vi "PH_StatusHandler.set GUI Refs.vi"(0 "i ref in":refnum<vi>, 1 "Class":string, 2 "GUI Ref":refnum<vi>, 3 "Blinking (false)":bool, 4 "Tip Strip":string="N/A", 5 "error in (no error)":errorcluster) -> (14 "i ref out":refnum<vi>, 19 "error out":errorcluster)   [LabVIEW 2014, in "PH_StatusHandler.lvlib"]
doc: "By this VI the GUI refs are stored to own attributes."
uses:
  PH_StatusHandler.lvlib
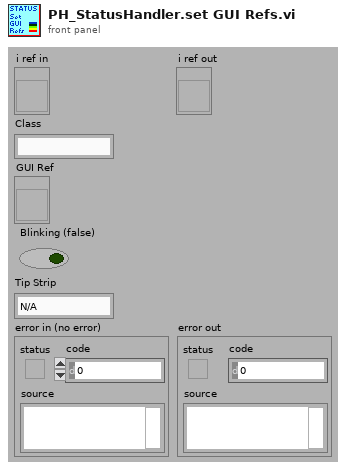
[diagram p1: front panel]
types:
  T1 = typedef "PH_StatusHandler.lvlib/PH_StatusHandler.i attribute.ctl" = cluster{"GUI Ref":refnum<vi>, "Value":T2, "Service ID":i32}
  T2 = typedef "PH_StatusHandler.lvlib/PH_StatusHandler.Status.ctl" = i16
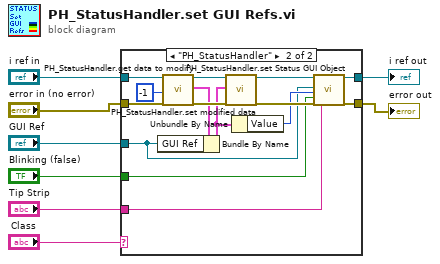
[diagram p0: block diagram]
diagram:
  n1 = case shown="\"PH_StatusHandler\"" "Class" {
    tunnel: "i ref in" -> [w10 w24]
    tunnel: "error in (no error)" -> [w9 w23]
    tunnel: "GUI Ref" -> [_ w13]
    tunnel: [w10 w18] -> w5
    tunnel: [w9 w16] -> w4
    tunnel: "Blinking (false)" -> [_ w12]
    tunnel: "Tip Strip" -> [_ w11]
    frame Default {
    }
    frame "PH_StatusHandler" {
      n2 = call "PH_StatusHandler.get data to modify.vi"("i ref in"=w24, "ms timeout (10000)"=-1, "error in (no error)"=w23) -> ("i ref out"=w20:refnum<vi>, "i attribute"=w21:T1, "error out"=w22:errorcluster)  [unwired: 13 in, 1 out]
      n3 = Bundle By Name(cluster=w21, "GUI Ref"=w13) -> (w15:T1)
      n4 = call "PH_StatusHandler.set modified data.vi"("i ref in"=w20, "i attribute"=w15, "error in (no error)"=w22) -> ("i ref out"=w18:refnum<vi>, "error out"=w17:errorcluster)  [unwired: 15 in]
      n5 = Unbundle By Name(w15) -> ("Value"=w14:T2)
      n6 = call "PH_StatusHandler.set Status GUI Object.vi"("PH Status Ref"=w13, "Value"=w14, "Blinking (false)"=w12, "error in (no error)"=w17, "Tip Strip"=w11) -> ("error out"=w16:errorcluster)  [unwired: 14 in]
    }
  }
  "i ref out" <- w5
  "error out" <- w4
